vi "computeReward.vi"(0 "RewardedLength":refnum<vi>, 1 "X":refnum<vi>, 2 "Y":refnum<vi>, 3 "TrialListElements":T1, 5 "targpos":dbl[](array[numeric])) -> (7 "ylen":dbl, 8 "completed":bool, 9 "reward":dbl, 10 "xlen":dbl)   [LabVIEW 2018]
uses:
  TrialListElements.ctl
  trial type.ctl
  rewtype.ctl
  <vilib>/imath/engines/lvmath2/RunTimeEngine/RunTimeType/NIMS_RunTimeType_From StrictType (excl LVString).vi
  <instcachedir>/0/NIMS_RunTimeType_From StrictType (excl LVString)_E7E34A65C99947108168652BAD14964D.lvgen/NIMS_RunTimeType_From StrictType (excl LVString)_E7E34A65C99947108168652BAD14964D_050.vi
  <instcachedir>/0/NIMS_RunTimeType_From StrictType (excl LVString)_E7E34A65C99947108168652BAD14964D.lvgen/NIMS_RunTimeType_From StrictType (excl LVString)_E7E34A65C99947108168652BAD14964D_032.vi
  <instcachedir>/0/NIMS_RunTimeType_From StrictType (excl LVString)_E7E34A65C99947108168652BAD14964D.lvgen/NIMS_RunTimeType_From StrictType (excl LVString)_E7E34A65C99947108168652BAD14964D_031.vi
  <instcachedir>/0/NIMS_RunTimeType_From StrictType (excl LVString)_E7E34A65C99947108168652BAD14964D.lvgen/NIMS_RunTimeType_From StrictType (excl LVString)_E7E34A65C99947108168652BAD14964D_049.vi
  <vilib>/imath/engines/lvmath2/RunTimeEngine/Struct/NIMS_StructSetField.vi
  <vilib>/imath/engines/lvmath2/RunTimeEngine/Struct/NIMS_StructGetField.vi
  <vilib>/imath/engines/lvmath2/RunTimeEngine/RunTimeType/NIMS_RunTimeType_To Numeric.vi
  <instcachedir>/0/NIMS_RunTimeType_To Numeric_56D9B3D2177F45D4A08165E143DC65A4.lvgen/NIMS_RunTimeType_To Numeric_56D9B3D2177F45D4A08165E143DC65A4_008.vi
  <vilib>/imath/engines/lvmath2/RunTimeEngine/ArithmeticOperatorToken/NIMS_ArithmeticOperator_multmx(M,CV)-internal.vi
  <instcachedir>/0/NIMS_ArithmeticOperator_multmx(M,CV)-internal_5287250D8D1D4A3E9F77F5DF08D432E0.lvgen/NIMS_ArithmeticOperator_multmx(M,CV)-internal_5287250D8D1D4A3E9F77F5DF08D432E0_002.vi
  <vilib>/imathl/engines/lvmath/Functions/Error Handling/Create Error.vi
  <vilib>/imath/engines/lvmath2/RunTimeEngine/IndexRead/NIMS V(S).vi
  <instcachedir>/0/NIMS V(S)_0488751826AF41519A22953C041130DC.lvgen/NIMS V(S)_0488751826AF41519A22953C041130DC_000.vi
  <instcachedir>/0/NIMS_RunTimeType_To Numeric_56D9B3D2177F45D4A08165E143DC65A4.lvgen/NIMS_RunTimeType_To Numeric_56D9B3D2177F45D4A08165E143DC65A4_009.vi
  <vilib>/imath/engines/lvmath2/RunTimeEngine/BuiltInFunctions/abs/NIMS_abs(signed).vi
  <instcachedir>/0/NIMS_abs(signed)_C4FCB8E6058B49B797C7C8D53CA5F6EC.lvgen/NIMS_abs(signed)_C4FCB8E6058B49B797C7C8D53CA5F6EC_000.vi
  <vilib>/imath/engines/lvmath2/RunTimeEngine/VariableToken/NIMS_VariableToken_CondDefined.vi
  <instcachedir>/0/NIMS_VariableToken_CondDefined_BADDB804EBCA4B86883699DABD34B224.lvgen/NIMS_VariableToken_CondDefined_BADDB804EBCA4B86883699DABD34B224_004.vi
  <instcachedir>/0/NIMS_VariableToken_CondDefined_BADDB804EBCA4B86883699DABD34B224.lvgen/NIMS_VariableToken_CondDefined_BADDB804EBCA4B86883699DABD34B224_003.vi
  <vilib>/imath/engines/lvmath/Functions/Error Handling/MergeErrorsWrapper.vi
  <vilib>/imath/engines/lvmath2/RunTimeEngine/NodeEndStatement/NIMS_NodeEndStatement_Output.vi
  <instcachedir>/0/NIMS_NodeEndStatement_Output_53EC0D466D134D7ABD903AC30B43404B.lvgen/NIMS_NodeEndStatement_Output_53EC0D466D134D7ABD903AC30B43404B_010.vi
  <instcachedir>/0/NIMS_NodeEndStatement_Output_53EC0D466D134D7ABD903AC30B43404B.lvgen/NIMS_NodeEndStatement_Output_53EC0D466D134D7ABD903AC30B43404B_001.vi
  <vilib>/imath/engines/lvmath2/RunTimeEngine/ErrorHandling/NIMS_Finalize Error.vi
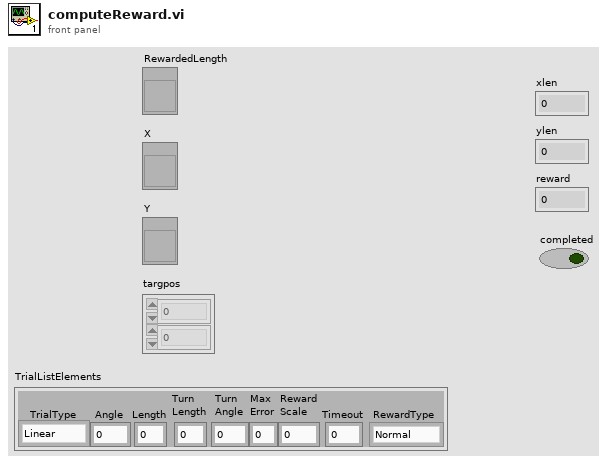
[diagram p1: front panel]
types:
  T1 = typedef "TrialListElements.ctl" = cluster{"TrialType":T2, "Angle":dbl, "Length":dbl, "TurnLength":dbl, "TurnAngle":dbl, "MaxError":dbl, "RewardScale":dbl, "Timeout":i32, "RewardType":T3}
  T2 = typedef "trial type.ctl" = enum8{"Linear", "2D aiming", "Two-part"}
  T3 = typedef "rewtype.ctl" = enum16{"Normal", "No reward"}
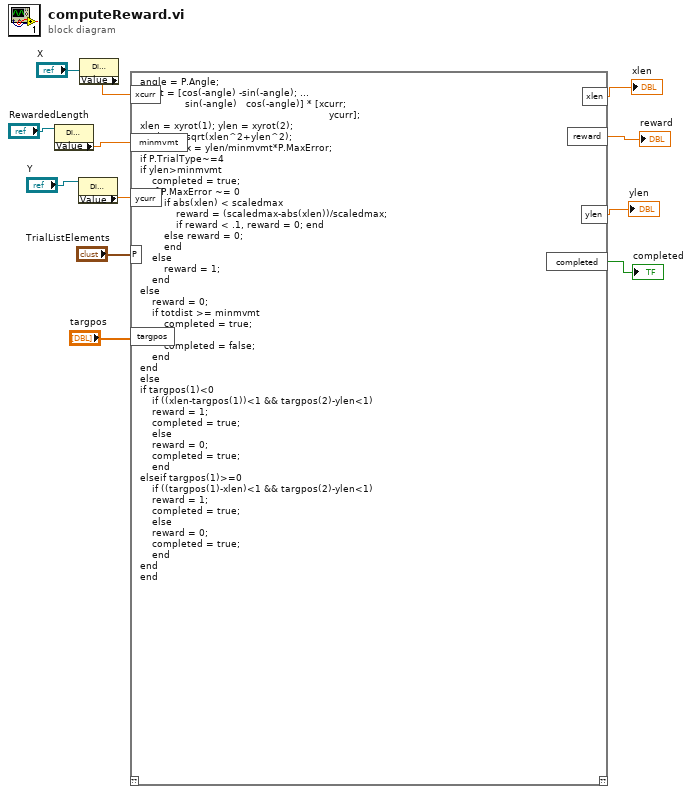
[diagram p0: block diagram]
diagram:
  n1 = property class="DigNum (strict)"(reference="RewardedLength") -> ("Value"=w12:sgl)  [unwired: 1 in, 2 out]
  n2 = property class="DigNum (strict)"(reference="Y") -> ("Value"=w10:sgl)  [unwired: 1 in, 2 out]
  n3 = property class="DigNum (strict)"(reference="X") -> ("Value"=w11:sgl)  [unwired: 1 in, 2 out]
  n4 = mathscript code="angle = P.Angle;\nxyrot = [cos(-angle) -sin(-angle); ...\n               sin(-angle)   cos(-angle)] * [xcurr;\n                                                               ycurr];\nxlen = xyrot(1); ylen = xyrot(2);\ntotdist = sqrt(xlen^2+ylen^2);\nscaledmax = ylen/minmvmt*P.MaxError;\nif P.TrialType~=4\nif ylen>minmvmt \n    completed = true;\n    if P.MaxError ~= 0\n        if abs(xlen) < scaledmax\n            reward = (scaledmax-abs(xlen))/scaledmax;\n            if reward < .1, reward = 0; end\n        else reward = 0;\n        end\n    else\n        reward = 1;\n    end\nelse \n    reward = 0;\n    if totdist >= minmvmt\n        completed = true;\n    else\n        completed = false;\n    end\nend\nelse\nif targpos(1)<0\n    if ((xlen-targpos(1))<1 && targpos(2)-ylen<1)\n    reward = 1;\n    completed = true;\n    else\n    reward = 0;\n    completed = true;\n    end\nelseif targpos(1)>=0\n    if ((targpos(1)-xlen)<1 && targpos(2)-ylen<1)\n    reward = 1;\n    completed = true;\n    else\n    reward = 0;\n    completed = true;\n    end\nend\nend"("ycurr"=w10, "xcurr"=w11, "P"="TrialListElements", "minmvmt"=w12, "targpos"="targpos") -> ("xlen"=→"xlen":dbl, "ylen"=→"ylen":dbl, "reward"=→"reward":dbl, "completed"=→"completed":bool)  [unwired: 1 in, 1 out]
